vi "Module Execution Decimation.vi"(11 "Module Info In":T1) -> (3 "Module Info Out":T1)   [LabVIEW 2013]
uses:
  Module Execution Info.ctl
  <vilib>/NI/Tag Bus Module Framework/runtime/TBM module execution interface.lvclass
  Data Table with Transfer Spec.ctl
  <vilib>/NI/Tag Bus/table/data table.ctl
  <vilib>/NI/Tag Bus/table/transfer specification.ctl
  <vilib>/NI/Tag Bus/tag/Data Type.ctl
  Configuration/Module Decimation.ctl
  Configuration/Module Error Configuration.ctl
  Configuration/Error Actions By Category.ctl
  <vilib>/NI/Tag Bus Module Framework/runtime/error classification.ctl
  Configuration/Error Actions.ctl
  error responses.ctl
  Configuration/error options.ctl
  Configuration/Standard Engine Configuration.lvclass
  <vilib>/NI/Tag Bus/tag/tag descriptor.lvclass
  <vilib>/NI/Tag Bus/table/data table.lvlib
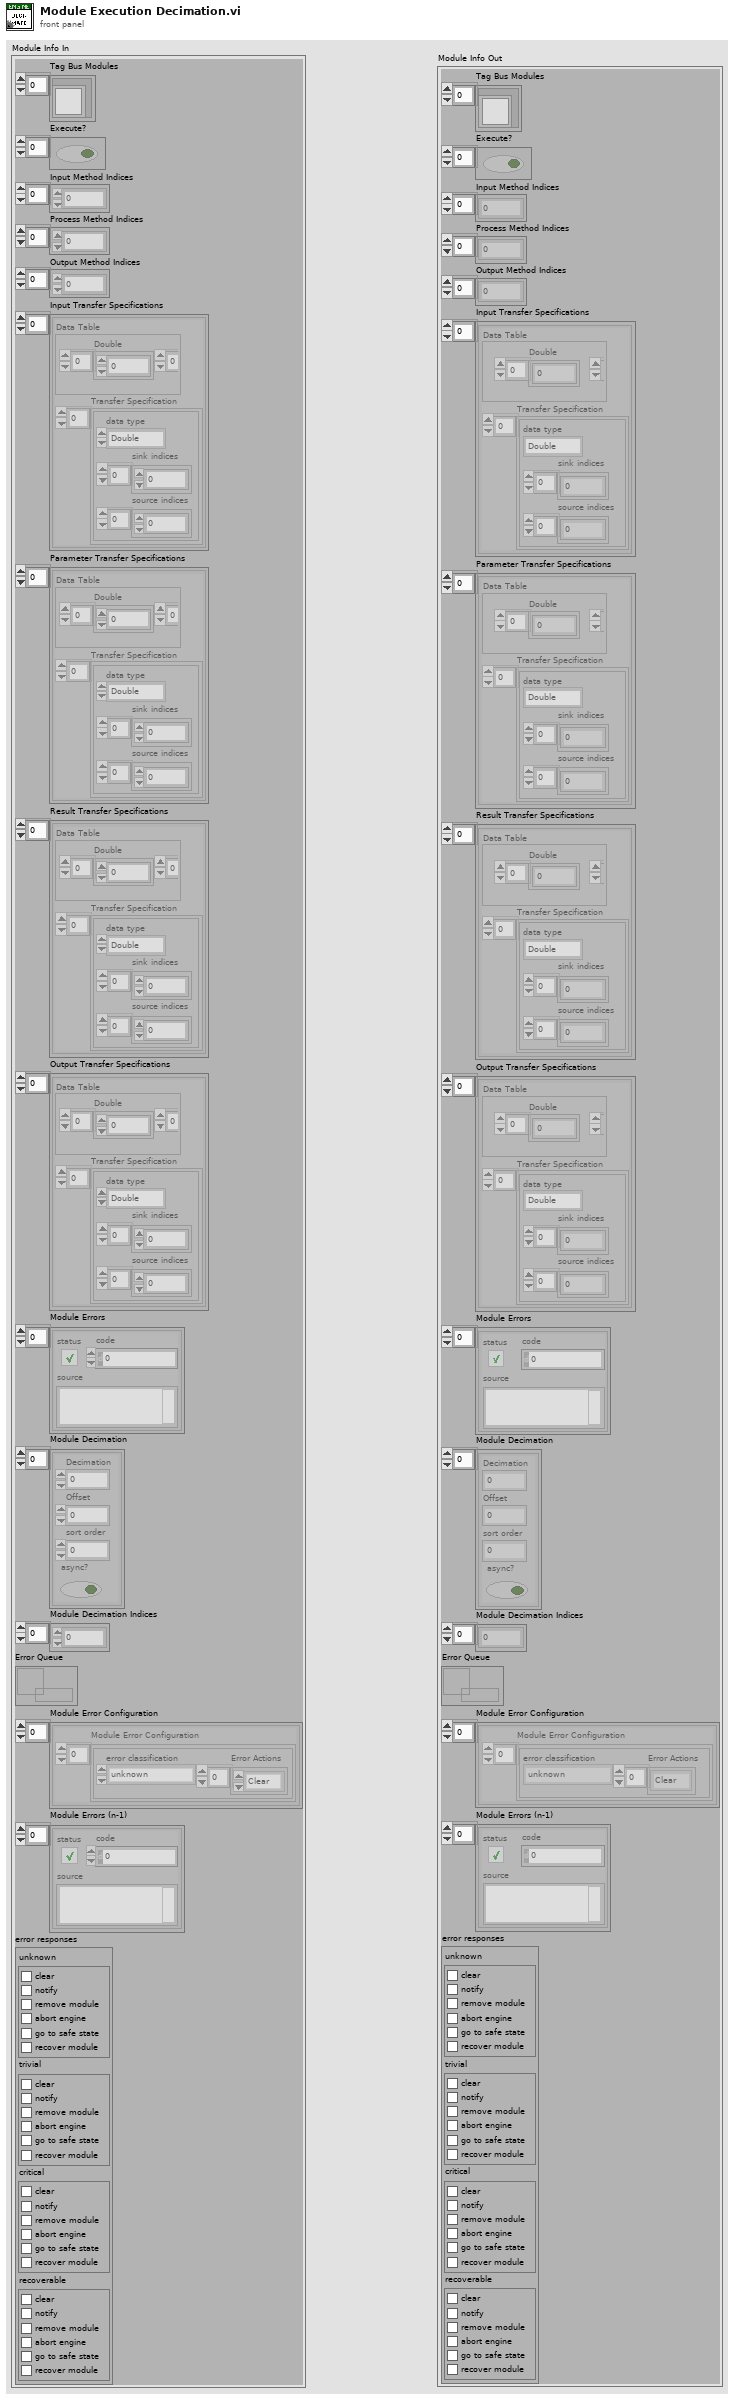
[diagram p1: front panel]
types:
  T1 = typedef "Module Execution Info.ctl" = cluster{"Tag Bus Modules":refnum<class "TBM module execution interface.lvclass">[], "Execute?":bool[], "Input Method Indices":i32[], "Process Method Indices":i32[], "Output Method Indices":i32[], "Input Transfer Specifications":T2[], "Parameter Transfer Specifications":T2[], "Result Transfer Specifications":T2[], "Output Transfer Specifications":T2[], "Module Errors":errorcluster[], "Module Decimation":T6[], "Module Decimation Indices":i32[], "Error Queue":refnum<queue>, "Module Error Configuration":T7[], "Module Errors (n-1)":errorcluster[], "error responses":T11}
  T2 = typedef "Data Table with Transfer Spec.ctl" = cluster{"Data Table":T3, "Transfer Specification":T4[]}
  T3 = typedef "tag bus.lvlib/data table.lvlib/data table.ctl" = cluster{"Double":dbl[], "Single":sgl[], "I64":i64[], "I32":i32[], "I16":i16[], "I8":i8[], "U64":u64[], "U32":u32[], "U16":u16[], "U8":u8[], "Boolean":bool[], "String":string[], "Array of Double":cluster{"DBL Array":dbl[]}[], "Array of Single":cluster{"SGL Array":sgl[]}[], "Array of I64":cluster{"I64 Array":i64[]}[], "Array of I32":cluster{"I32 Array":i32[]}[], "Array of I16":cluster{"I16 Array":i16[]}[], "Array of I8":cluster{"I8 Array":i8[]}[], "Array of U64":cluster{"U64 Array":u64[]}[], "Array of U32":cluster{"U32 Array":u32[]}[], "Array of U16":cluster{"U16 Array":u16[]}[], "Array of U8":cluster{"U8 Array":u8[]}[], "Array of Boolean":cluster{"Boolean Array":bool[]}[], "Array of String":cluster{"String Array":string[]}[]}
  T4 = typedef "tag bus.lvlib/data table.lvlib/transfer specification.ctl" = cluster{"data type":T5, "sink indices":i32[], "source indices":i32[]}
  T5 = typedef "tag bus.lvlib/tag descriptor.lvclass/Data Type.ctl" = enum16{"Double", "Single", "I64", "I32", "I16", "I8", "U64", "U32", "U16", "U8", "Boolean", "String", "Array of Double", "Array of Single", "Array of I64", "Array of I32", "Array of I16", "Array of I8", "Array of U64", "Array of U32", "Array of U16", "Array of U8", "Array of Boolean", "Array of String"}
  T6 = typedef "Standard Engine Configuration.lvclass/Module Decimation.ctl" = cluster{"Decimation":u16, "Offset":u16, "sort order":i32, "async?":bool}
  T7 = typedef "Standard Engine Configuration.lvclass/Module Error Configuration.ctl" = cluster{"Module Error Configuration":T8[]}
  T8 = typedef "Standard Engine Configuration.lvclass/Error Actions By Category.ctl" = cluster{"error classification":T9, "Error Actions":T10[]}
  T9 = typedef "TBM module execution interface.lvclass/error classification.ctl" = enum16{"unknown", "none", "trivial", "recoverable", "critical"}
  T10 = typedef "Standard Engine Configuration.lvclass/Error Actions.ctl" = enum16{"Clear", "Notify", "Stop Component", "Stop Engine", "Safe State", "Attempt Recovery"}
  T11 = typedef "Standard Engine Configuration.lvclass/error responses.ctl" = cluster{"unknown":T12, "trivial":T12, "critical":T12, "recoverable":T12}
  T12 = typedef "Standard Engine Configuration.lvclass/error options.ctl" = cluster{"clear":bool, "notify":bool, "remove module":bool, "abort engine":bool, "go to safe state":bool, "recover module":bool}
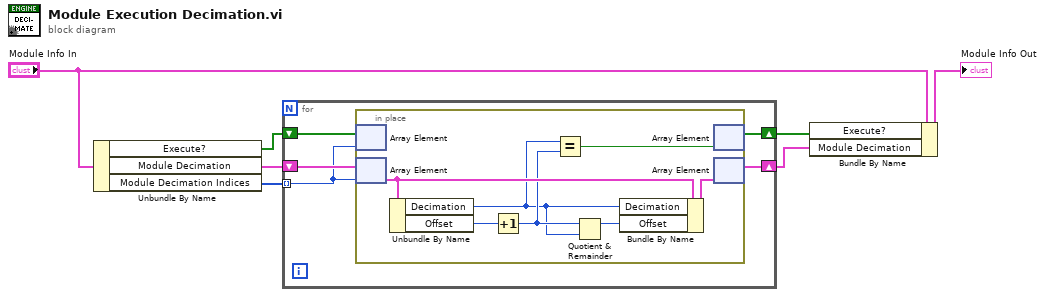
[diagram p0: block diagram]
diagram:
  n1 = Unbundle By Name("Module Info In") -> ("Execute?"=w7:bool[], "Module Decimation"=w6:T6[], "Module Decimation Indices"=w5:i32[])
  n2 = for {
    tunnel: w5 -> [w8] mode=indexing
    shift-right: [w10] -> w3
    shift-left: w7 -> [w11]
    shift-right: [w9] -> w2
    shift-left: w6 -> [w12]
    n3 = in-place {
      n4 = in-place-array #1(w11, w8) -> ()  [unwired: 1 out]
      n5 = in-place-array #2(w12, w8) -> (w19:T6)
      n6 = Unbundle By Name(w19) -> ("Decimation"=w15:u16, "Offset"=w18:u16)
      n7 = Increment(x=w18) -> (x+1=w16:u16)
      n8 = Equal?(x=w15, y=w16) -> (x = y?=w13:bool)
      n9 = Quotient & Remainder(x=w16, y=w15) -> (x-y*floor(x/y)=w14:u16)  [unwired: 1 out]
      n10 = Bundle By Name(cluster=w19, "Decimation"=w15, "Offset"=w14) -> (w17:T6)
      n11 = in-place-array #1(w13) -> (w10:bool[])  [unwired: 1 out]
      n12 = in-place-array #2(w17) -> (w9:T6[])  [unwired: 1 out]
    }
  }
  n13 = Bundle By Name(cluster="Module Info In", "Execute?"=w3, "Module Decimation"=w2) -> (→"Module Info Out":T1)
